vi "MyTest.vi"() -> ()   [LabVIEW 2017]
uses:
  Intake/Implementation/Intake Setpoints.ctl
  Intake/Implementation/Intake Operations.ctl
  <vilib>/Rock Robotics/WPI/Framework/Completion Status.ctl
  <vilib>/Rock Robotics/SystemInterfaces/AI/FPGA_AIChannel.ctl
  <vilib>/Rock Robotics/SystemInterfaces/DIO/FPGA_DIOPWMChannel.ctl
  <vilib>/Rock Robotics/WPI/SafetyOutput/WPI_SafetyOutputConfigMenu.ctl
  <vilib>/Rock Robotics/WPI/MotorControl/WPI_MotorControlOpen SPARK.vi
  LabVIEW Data/TestProject/Intake/Implementation/Degree Setpoint Global.vi
  <vilib>/Rock Robotics/Network Tables/NT Write Boolean.vi
panel:
  in  "Degree Setpoint":dbl(slide) scale=0.0..1.0
  in  "Buttons":cluster{"Execute Cmd":bool, "Abort Cmd":bool}
  out "Status":T1
  out "Command Timing":cluster{"Start Time (ms)":u32, "Iterations":i32}
  in  "Interactive Values":T2
  out "Numeric":i32
  in  "error in":errorcluster
  out "Boolean":bool=TRUE
  in  "haveCube (sensor)":bool
  out "Current\nCmd":string
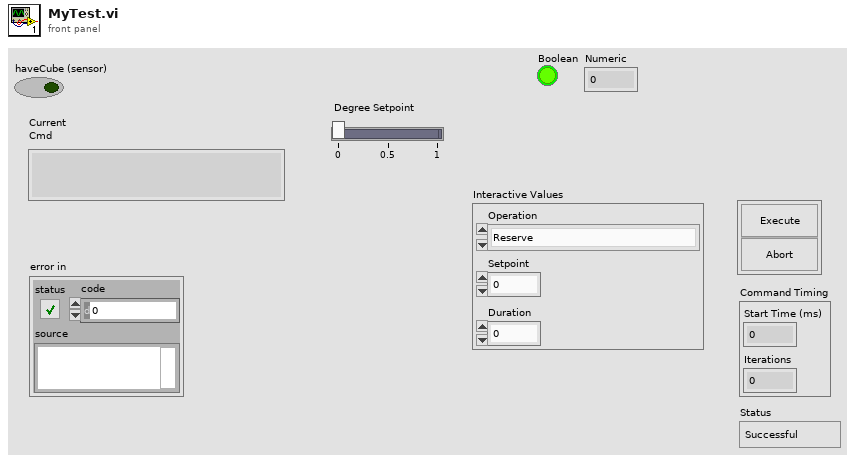
[diagram p1: front panel]
types:
  T1 = typedef "Completion Status.ctl" = enum16{"Successful", "Aborted", "Incomplete"}
  T2 = typedef "Intake Setpoints.ctl" = cluster{"Operation":T3, "Setpoint":dbl, "Duration":dbl}
  T3 = typedef "Intake Operations.ctl" = enum16{"Reserve", "Read Current", "setSetpoint", "feed", "spit"}
  T4 = typedef "FPGA_AIChannel.ctl" = enum8{"AI 0", "AI 1", "AI 2", "AI 3", "AI MXP 0", "AI MXP 1", "AI MXP 2", "AI MXP 3", "Invalid"}
  T5 = typedef "WPI_PotentiometerDevRef.ctl" = cluster{"DevStatus":errorcluster, "Analog Channel":T4, "Invert Output":bool}
  T6 = typedef "WPI_SafetyOutputConfigMenu.ctl" = enum16{"Enable", "Disable"}
  T7 = typedef "FPGA_DIOPWMChannel.ctl" = enum8{"PWM 0", "PWM 1", "PWM 2", "PWM 3", "PWM 4", "PWM 5", "PWM 6", "PWM 7", "PWM 8", "PWM 9", "PWM MXP 0", "PWM MXP 1", "PWM MXP 2", "PWM MXP 3", "PWM MXP 4", "PWM MXP 5", "PWM MXP 6", "PWM MXP 7", "PWM MXP 8", "PWM MXP 9", "Invalid"}
  T8 = typedef "WPI_MotorControlDeviceRef.ctl" = cluster{"DeviceStatus":errorcluster, "Type":T9, "PWM":cluster{"PWM Channel":T7, "DeadBand":T10}, "CAN":cluster{"Device Number":u8, "SetOutput VI Ref":variant, "GetOutput VI Ref":variant, "Enable VI Ref":variant, "Disable VI Ref":variant, "Data":variant}, "Invert":bool, "DIO PWM":cluster{"PWM \"Enable\" Channel":T7, "DIOChannel":T11, "PWM Rate":dbl}}
  T9 = typedef "WPI_MotorControlType.ctl" = enum16{"PWM", "CAN", "DIO PWM"}
  T10 = typedef "WPI_PWMDeadband.ctl" = cluster{"Name":string, "maxPositivePwm":i32, "minPositivePwm":i32, "centerPwm":i32, "maxNegativePwm":i32, "minNegativePwm":i32, "angularRange":u16}
  T11 = typedef "FPGA_DIOChannel.ctl" = enum8{"DIO 0", "DIO 1", "DIO 2", "DIO 3", "DIO 4", "DIO 5", "DIO 6", "DIO 7", "DIO 8", "DIO 9", "DIO MXP 0", "DIO MXP 1", "DIO MXP 2", "DIO MXP 3", "DIO MXP 4", "DIO MXP 5", "DIO MXP 6", "DIO MXP 7", "DIO MXP 8", "DIO MXP 9", "DIO MXP 10", "DIO MXP 11", "DIO MXP 12", "DIO MXP 13", "DIO MXP 14", "DIO MXP 15", "SPI Port CS1", "SPI Port CS2", "SPI Port CS3", "SPI Port MISO", "SPI Port MOSI", "Invalid"}
  T12 = typedef "Command Status Info.ctl" = cluster{"Name":string, "Status":T1, "notifier out":T13}
  T13 = typedef "Completion Notifier.ctl" = refnum<notifier>
  T14 = cluster{"Current Command":T2, "Command Timing":cluster{"Start Time (ms)":u32, "Iterations":i32}, "Command Arguments":cluster{"Command Info":T12, "Description":string, "Default Command":T2, "queue out":refnum<queue>, "Subsystem Name":string}}
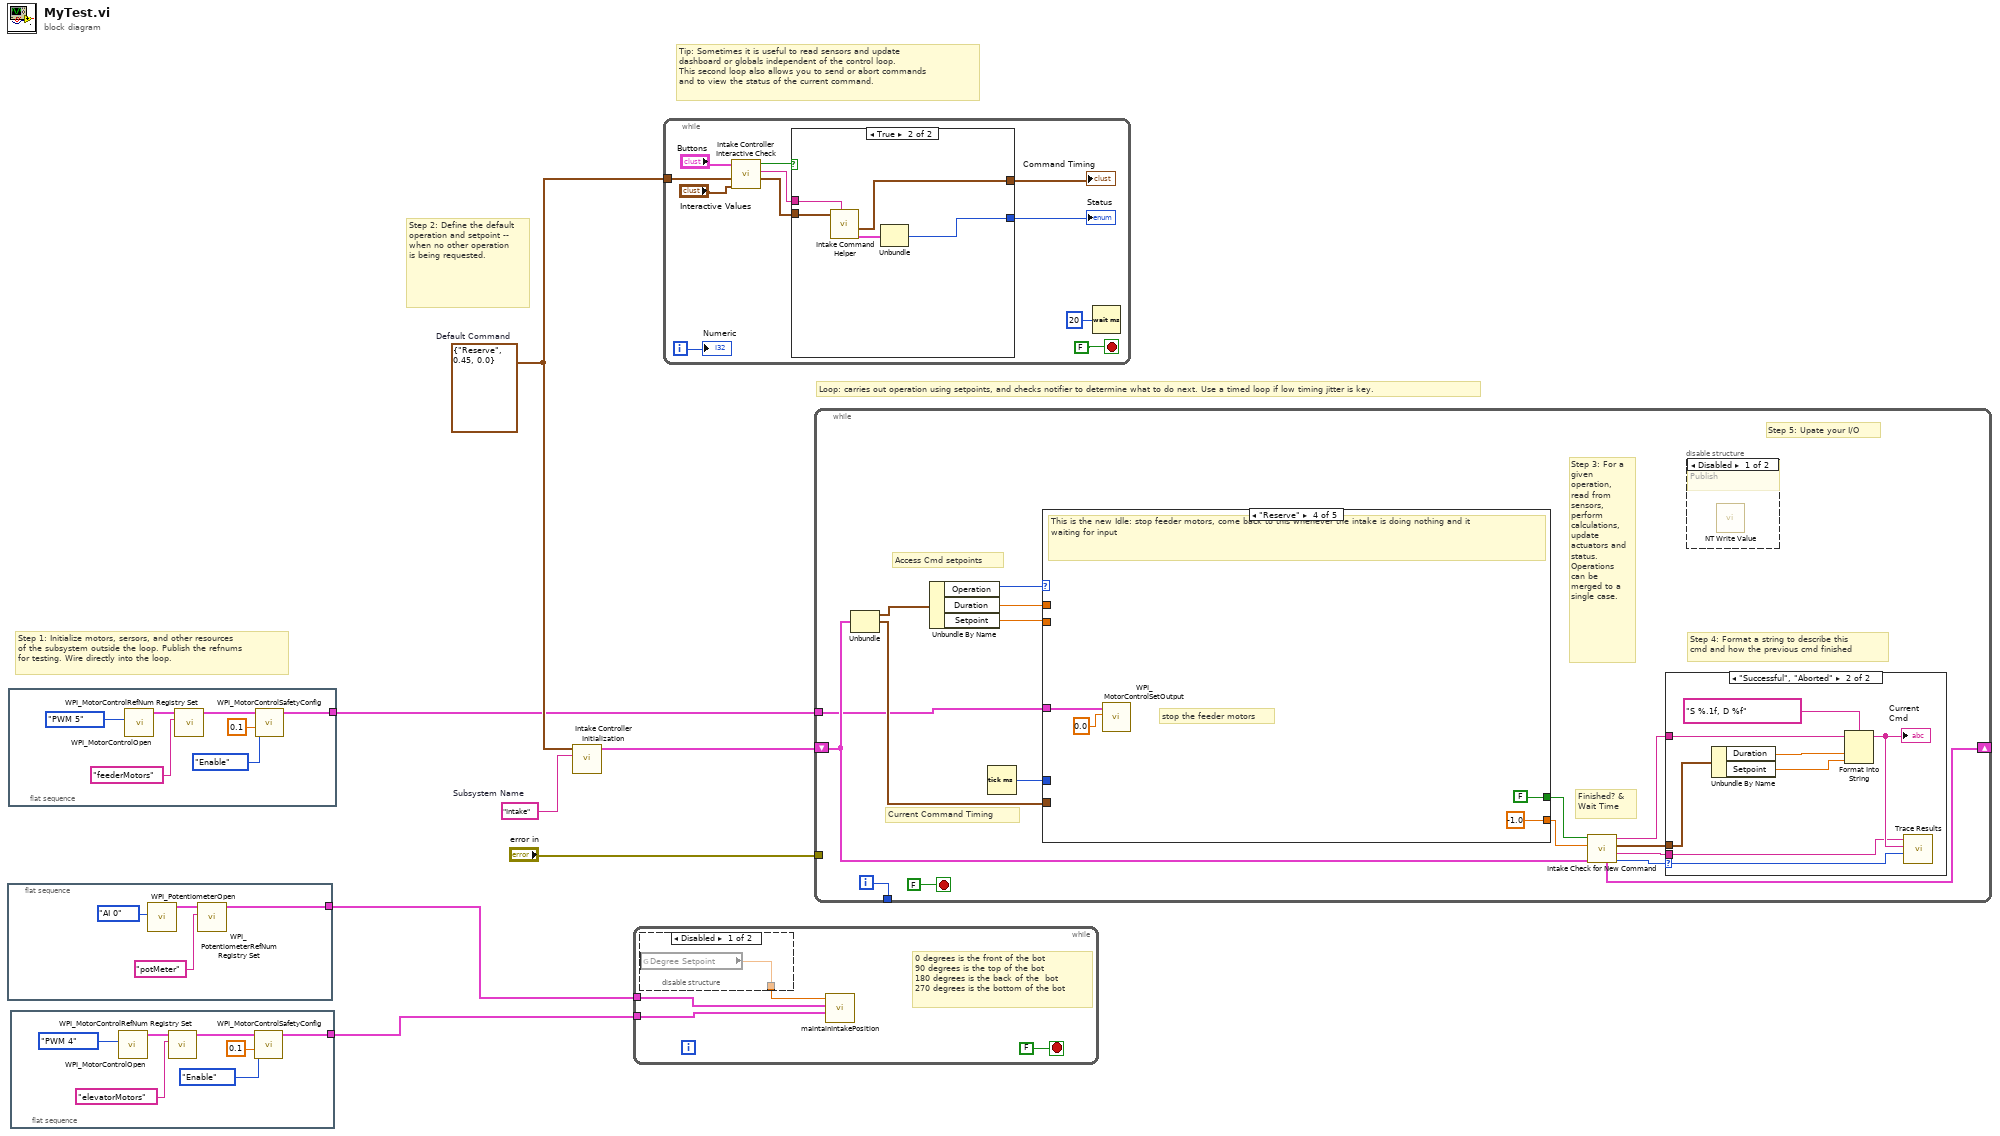
[diagram p0: block diagram]
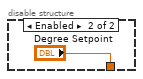
[diagram p2: hidden frame]
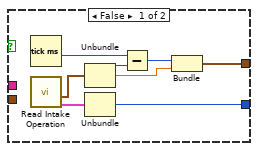
[diagram p3: hidden frame]
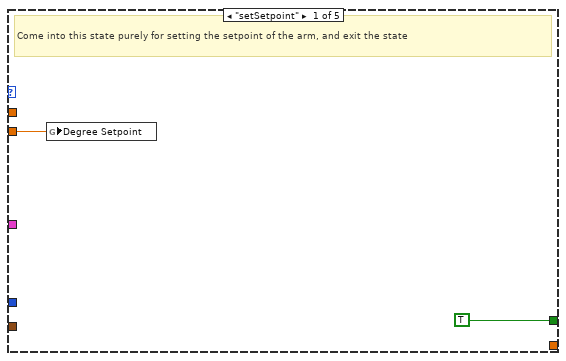
[diagram p6: hidden frame]
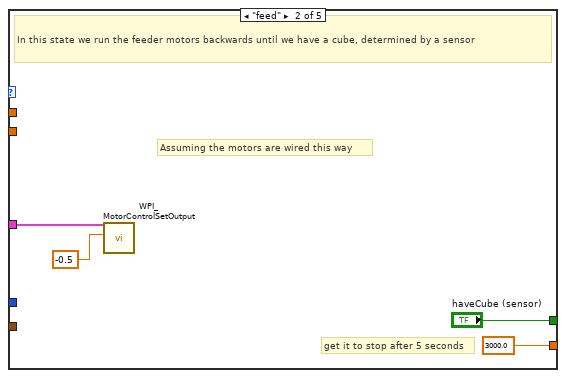
[diagram p7: hidden frame]
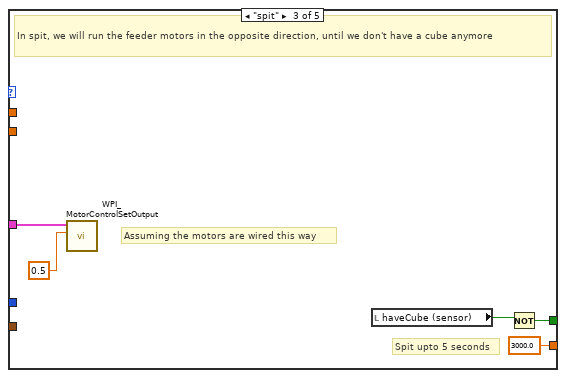
[diagram p8: hidden frame]
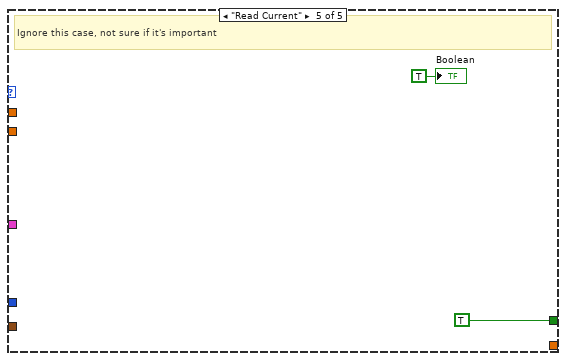
[diagram p9: hidden frame]
diagram:
  w4 = T2 {"Operation"=enum."Reserve", "Setpoint"=0.45, "Duration"=0.0}  # Default Command
  w5 = "Intake"  # Subsystem Name
  # "Tip: Sometimes it is useful to read sensors and update\ndashboard or globals independent of the control loop.\nThis second loop also allows you to send or abort commands\nand to view the status of the current command."
  # "Step 2: Define the default operation and setpoint --\nwhen no other operation is being requested."
  # "Step 1: Initialize motors, sersors, and other resources\nof the subsystem outside the loop. Publish the refnums\nfor testing. Wire directly into the loop."
  # "Loop: carries out operation using setpoints, and checks notifier to determine what to do next. Use a timed loop if low timing jitter is key."
  n1 = flat-sequence {
    tunnel: [w8] -> w1
    frame #0 {
      n2 = call <vilib>:"WPI_PotentiometerOpen.vi"("Analog Channel"=FPGA_AIChannel."AI 0") -> ("PotDevRef"=w9:T5)  [unwired: 9 in, 1 out]
      n3 = call <vilib>:"WPI_PotentiometerRefNum Registry Set.vi"("refnum name"="potMeter", "PotDevRef"=w9) -> ("PotDevRef"=w8:T5)  [unwired: 8 in, 1 out]
    }
  }
  n4 = flat-sequence {
    tunnel: [w14] -> w3
    frame #0 {
      n5 = call-poly <vilib>:"WPI_MotorControlOpen.vi"("PWM Channel"=FPGA_DIOPWMChannel."PWM 5") -> ("MotorControlDeviceRef"=w17:T8)  [unwired: 9 in, 1 out]
      n6 = call <vilib>:"WPI_MotorControlRefNum Registry Set.vi"("refnum name"="feederMotors", "MotorControlDevRef"=w17) -> ("MotorControlDevRef"=w15:T8)  [unwired: 8 in, 1 out]
      n7 = call <vilib>:"WPI_MotorControlSafetyConfig.vi"("timeout (s)"=0.1, "mode"=WPI_SafetyOutputConfigMenu."Enable", "MotorControlDevRef"=w15) -> ("MotorControlDevRef"=w14:T8)  [unwired: 7 in, 1 out]
    }
  }
  n8 = flat-sequence {
    tunnel: [w21] -> w2
    frame #0 {
      n9 = call-poly <vilib>:"WPI_MotorControlOpen.vi"("PWM Channel"=FPGA_DIOPWMChannel."PWM 4") -> ("MotorControlDeviceRef"=w24:T8)  [unwired: 9 in, 1 out]
      n10 = call <vilib>:"WPI_MotorControlRefNum Registry Set.vi"("refnum name"="elevatorMotors", "MotorControlDevRef"=w24) -> ("MotorControlDevRef"=w22:T8)  [unwired: 8 in, 1 out]
      n11 = call <vilib>:"WPI_MotorControlSafetyConfig.vi"("timeout (s)"=0.1, "mode"=WPI_SafetyOutputConfigMenu."Enable", "MotorControlDevRef"=w22) -> ("MotorControlDevRef"=w21:T8)  [unwired: 7 in, 1 out]
    }
  }
  n12 = call "Intake Controller Initialization.vi"("Subsystem Name"=w5, "Default Command"=w4) -> ("Current Command"=w6:T14)  [unwired: 9 in]
  n13 = while {
    tunnel: w2 -> [w28]
    tunnel: w1 -> [w27]
    stop <- FALSE stop-if-true
    # "0 degrees is the front of the bot\n90 degrees is the top of the bot\n180 degrees is the back of the  bot\n270 degrees is the bottom of the bot"
    n14 = disable-structure shown="Disabled" {
      disable-tunnel: [w30 "Degree Setpoint"] -> w26
      frame Disabled {
        n15 = global read "Degree Setpoint Global.vi" "Degree Setpoint"() -> (w30:dbl)
      }
      frame Enabled {
      }
    }
    n16 = call "maintainIntakePosition.vi"("MotorControlDevRef"=w28, "PotDevRef"=w27, "Degree Setpoint"=w26) -> ()  [unwired: 8 in]
  }
  n17 = while {
    tunnel: w4 -> [w39]
    i -> [w32]
    stop <- FALSE stop-if-true
    n18 = call "Intake Controller Interactive Check.vi"("Interactive Command in"="Interactive Values", "Default Command"=w39, "Buttons"="Buttons") -> ("Interactive Command out"=w36:T2, "Trace String"=w37:string, "Schedule"=w38:bool)  [unwired: 6 in]
    n19 = case shown="True" w38 {
      tunnel: [w50 w55] -> w35
      tunnel: w36 -> [_ w53]
      tunnel: [w46 w51] -> w34
      tunnel: w37 -> [_ w54]
      frame False {
        n20 = Tick Count (ms)() -> (millisecond timer value=w45:u32)
        n21 = call "Read Intake Operation.vi"() -> ("Command Info"=w43:T12, "SubSystem Data"=w44:T2)  [unwired: 9 in, 1 out]
        n22 = Unbundle(w44) -> ("Operation"=w49:T3, "Setpoint"=w47:dbl)  [unwired: 1 out]
        n23 = Unbundle(w43) -> ("Status"=w50:T1)  [unwired: 2 out]
        n24 = Subtract(x=w45, y=w49) -> (x-y=w48:u32)
        n25 = Bundle(w48, "Setpoint"=w47) -> (w46:cluster{u32, "Setpoint":dbl})  [unwired: 1 in]
      }
      frame True {
        n26 = call "Intake Command Helper.vi"("Description"=w54, "SubSystem Data"=w53) -> ("Command Info Out"=w52:T12, "Command Timing"=w51:cluster{"Start Time (ms)":u32, "Iterations":i32})  [unwired: 7 in, 1 out]
        n27 = Unbundle(w52) -> ("Status"=w55:T1)  [unwired: 2 out]
      }
    }
    "Status" <- w35
    "Command Timing" <- w34
    n28 = Wait (ms)(milliseconds to wait=u32 20) -> ()  [unwired: 1 out]
    "Numeric" <- w32
  }
  n29 = while {
    shift-right: [w64] -> _
    shift-left: w6 -> [w57]
    tunnel: [w71] -> _
    tunnel: "error in" -> [_]
    tunnel: w3 -> [w56]
    i -> [w71]
    stop <- FALSE stop-if-true
    # "Step 5: Upate your I/O"
    # "Step 4: Format a string to describe this\ncmd and how the previous cmd finished"
    # "Current Command Timing"
    # "Access Cmd setpoints"
    # "Finished? &\nWait Time"
    # "Step 3: For a given operation, read from sensors, perform calculations,\nupdate actuators and status.\nOperations can be merged to a single case."
    n30 = Unbundle(w57) -> ("Current Command"=w70:T2, "Command Timing"=w66:cluster{"Start Time (ms)":u32, "Iterations":i32})  [unwired: 1 out]
    n31 = Unbundle By Name(w70) -> ("Operation"=w69:T3, "Duration"=w68:dbl, "Setpoint"=w65:dbl)
    n32 = Tick Count (ms)() -> (millisecond timer value=w67:u32)
    n33 = case shown="\"Reserve\"" w69 {
      tunnel: [_ 3000.0 ("Infinite") 3000.0 ("Infinite") -1.0 ("Infinite") _] -> w62
      tunnel: [TRUE ("ignore previous (F)") "haveCube (sensor)" w88 FALSE ("ignore previous (F)") TRUE ("ignore previous (F)")] -> w63
      tunnel: w66 -> [_ _ _ _ _]
      tunnel: w68 -> [_ _ _ _ _]
      tunnel: w67 -> [_ _ _ _ _]
      tunnel: w65 -> [w81 _ _ _ _]
      tunnel: w56 -> [_ w86 w91 w93 _]
      frame "setSetpoint" {
        # "Come into this state purely for setting the setpoint of the arm, and exit the state"
        n34 = global write "Degree Setpoint Global.vi" "Degree Setpoint"(w81) -> ()
      }
      frame "feed" {
        # "get it to stop after 5 seconds"
        # "Assuming the motors are wired this way"
        # "In this state we run the feeder motors backwards until we have a cube, determined by a sensor"
        n35 = call <vilib>:"WPI_MotorControlSetOutput.vi"("Output"=-0.5, "MotorControlDevRef"=w86) -> ()  [unwired: 7 in, 3 out]
      }
      frame "spit" {
        # "Spit upto 5 seconds"
        # "Assuming the motors are wired this way"
        # "In spit, we will run the feeder motors in the opposite direction, until we don't have a cube anymore"
        n36 = call <vilib>:"WPI_MotorControlSetOutput.vi"("Output"=0.5, "MotorControlDevRef"=w91) -> ()  [unwired: 7 in, 3 out]
        n37 = local read "haveCube (sensor)"() -> (w87:bool)
        n38 = Not(x=w87) -> (.not. x?=w88:bool)
      }
      frame "Reserve" {
        # "stop the feeder motors"
        # "This is the new Idle: stop feeder motors, come back to this whenever the intake is doing nothing and it waiting for input"
        n39 = call <vilib>:"WPI_MotorControlSetOutput.vi"("Output"=0.0, "MotorControlDevRef"=w93) -> ()  [unwired: 7 in, 3 out]
      }
      frame "Read Current" {
        # "Ignore this case, not sure if it's important"
        "Boolean" <- TRUE
      }
    }
    n40 = call "Intake Check for New Command.vi"("Current Command"=w57, "Wait time (ms)"=w62, "Finished?"=w63) -> ("Completion"=w58:T1, "Subsystem Name"=w59:string, "Current Command"=w60:T2, "Initial Trace String"=w61:string, "NextCommand"=w64:T14)  [unwired: 4 in]
    n41 = case shown="\"Successful\", \"Aborted\"" w58 {
      selector: w58 -> [_ w80]
      tunnel: w61 -> [_ w76]
      tunnel: w60 -> [_ w77]
      tunnel: w59 -> [_ w73]
      frame "Incomplete", Default {
        # "Continuing current command"
      }
      frame "Successful", "Aborted" {
        # "Report and setup for next command"
        n42 = Unbundle By Name(w77) -> ("Duration"=w79:dbl, "Setpoint"=w74:dbl)
        n43 = Format Into String(format string="S %.1f, D %f", initial string=w76, w79, w74) -> (resulting string=w75:string)  [unwired: 1 in, 1 out]
        "Current\nCmd" <- w75
        n44 = call <vilib>:"Trace Results.vi"("Status of previous command"=w80, "Description"=w75, "Subsystem"=w73) -> ()  [unwired: 9 in]
      }
    }
    n45 = disable-structure shown="Disabled" {
      frame Disabled {
        # "Publish"
        n46 = call-poly <vilib>:"NT Write Value.vi"() -> ()  [unwired: 11 in, 1 out]
      }
      frame Enabled {
      }
    }
  }
